vi "Video Stuff v03.vi"() -> ()   [LabVIEW 2009]
doc: "This example illustrates the use of a calibration grid to calibrate and correct an image for nonlinear distortion and accurate shape measurements.\n\nThis example loads the image of a calibration grid used to calibrate the system, learns the grid, then loads an image of parts acquired using the same setup. The example then corrects the image in two ways. The first method corrects the entire image and then measures the area of the coins. The second method corrects only the area of the coins and displays the difference in processing time."
uses:
  <vilib>/userDefined/High Color/IMAQdx.ctl
  <vilib>/vision/NI_Vision_Development_Module.lvlib
  <vilib>/vision/driver/NI_Vision_Acquisition_Software.lvlib
panel:
  out "Image Pixels (U8)":u8[][](array[numeric])
  out "Array":i32[][](array[numeric])
  in  "Overlay":bool
  out "Small":T1(plugin-control)
  in  "Resolution":i32=36
  in  "Color":u32(colorbox)=16711885
  in  "Pixel Coordinates":cluster{"X":sgl, "Y":sgl}={"X"=146.5, "Y"=183.95} {"Y" format="%.2f"; "X" format="%.2f"}
  out "Real World Coordinates":cluster{"X":sgl, "Y":sgl} {"Y" format="%.2f"; "X" format="%.2f"}
  out "Transform":T1(plugin-control)
  in  "Camera Name":T2="cam0"
  in  "Video Modes":i32(listbox)
  in  "stop":bool
  out "Live Video":T1(plugin-control)
  out "Buffer Number":u32
  out "Frame Rate":dbl(knob) scale=0.0..100.0 scale format="%.1f"
  in  "Red Range":cluster{"Lower value":i32, "Upper value":i32}={"Lower value"=240, "Upper value"=255}
  in  "Green Range":cluster{"Lower value":i32, "Upper value":i32}={"Lower value"=250, "Upper value"=255}
  in  "Blue Range":cluster{"Lower value":i32, "Upper value":i32}={"Lower value"=250, "Upper value"=255}
  in  "Color Mode":u16(ring) items=["RGB", "HSL", "HSV", "HSI"]
  out "Super Filter":T1(plugin-control)
  in  "Calibration File Path":path=path "C:/Documents and Settings/ekolker/My Documents/OGRE/to be synched/calibrationGrid.PNG"
  out "Top Image":T1(plugin-control) caption="Calibration Template"
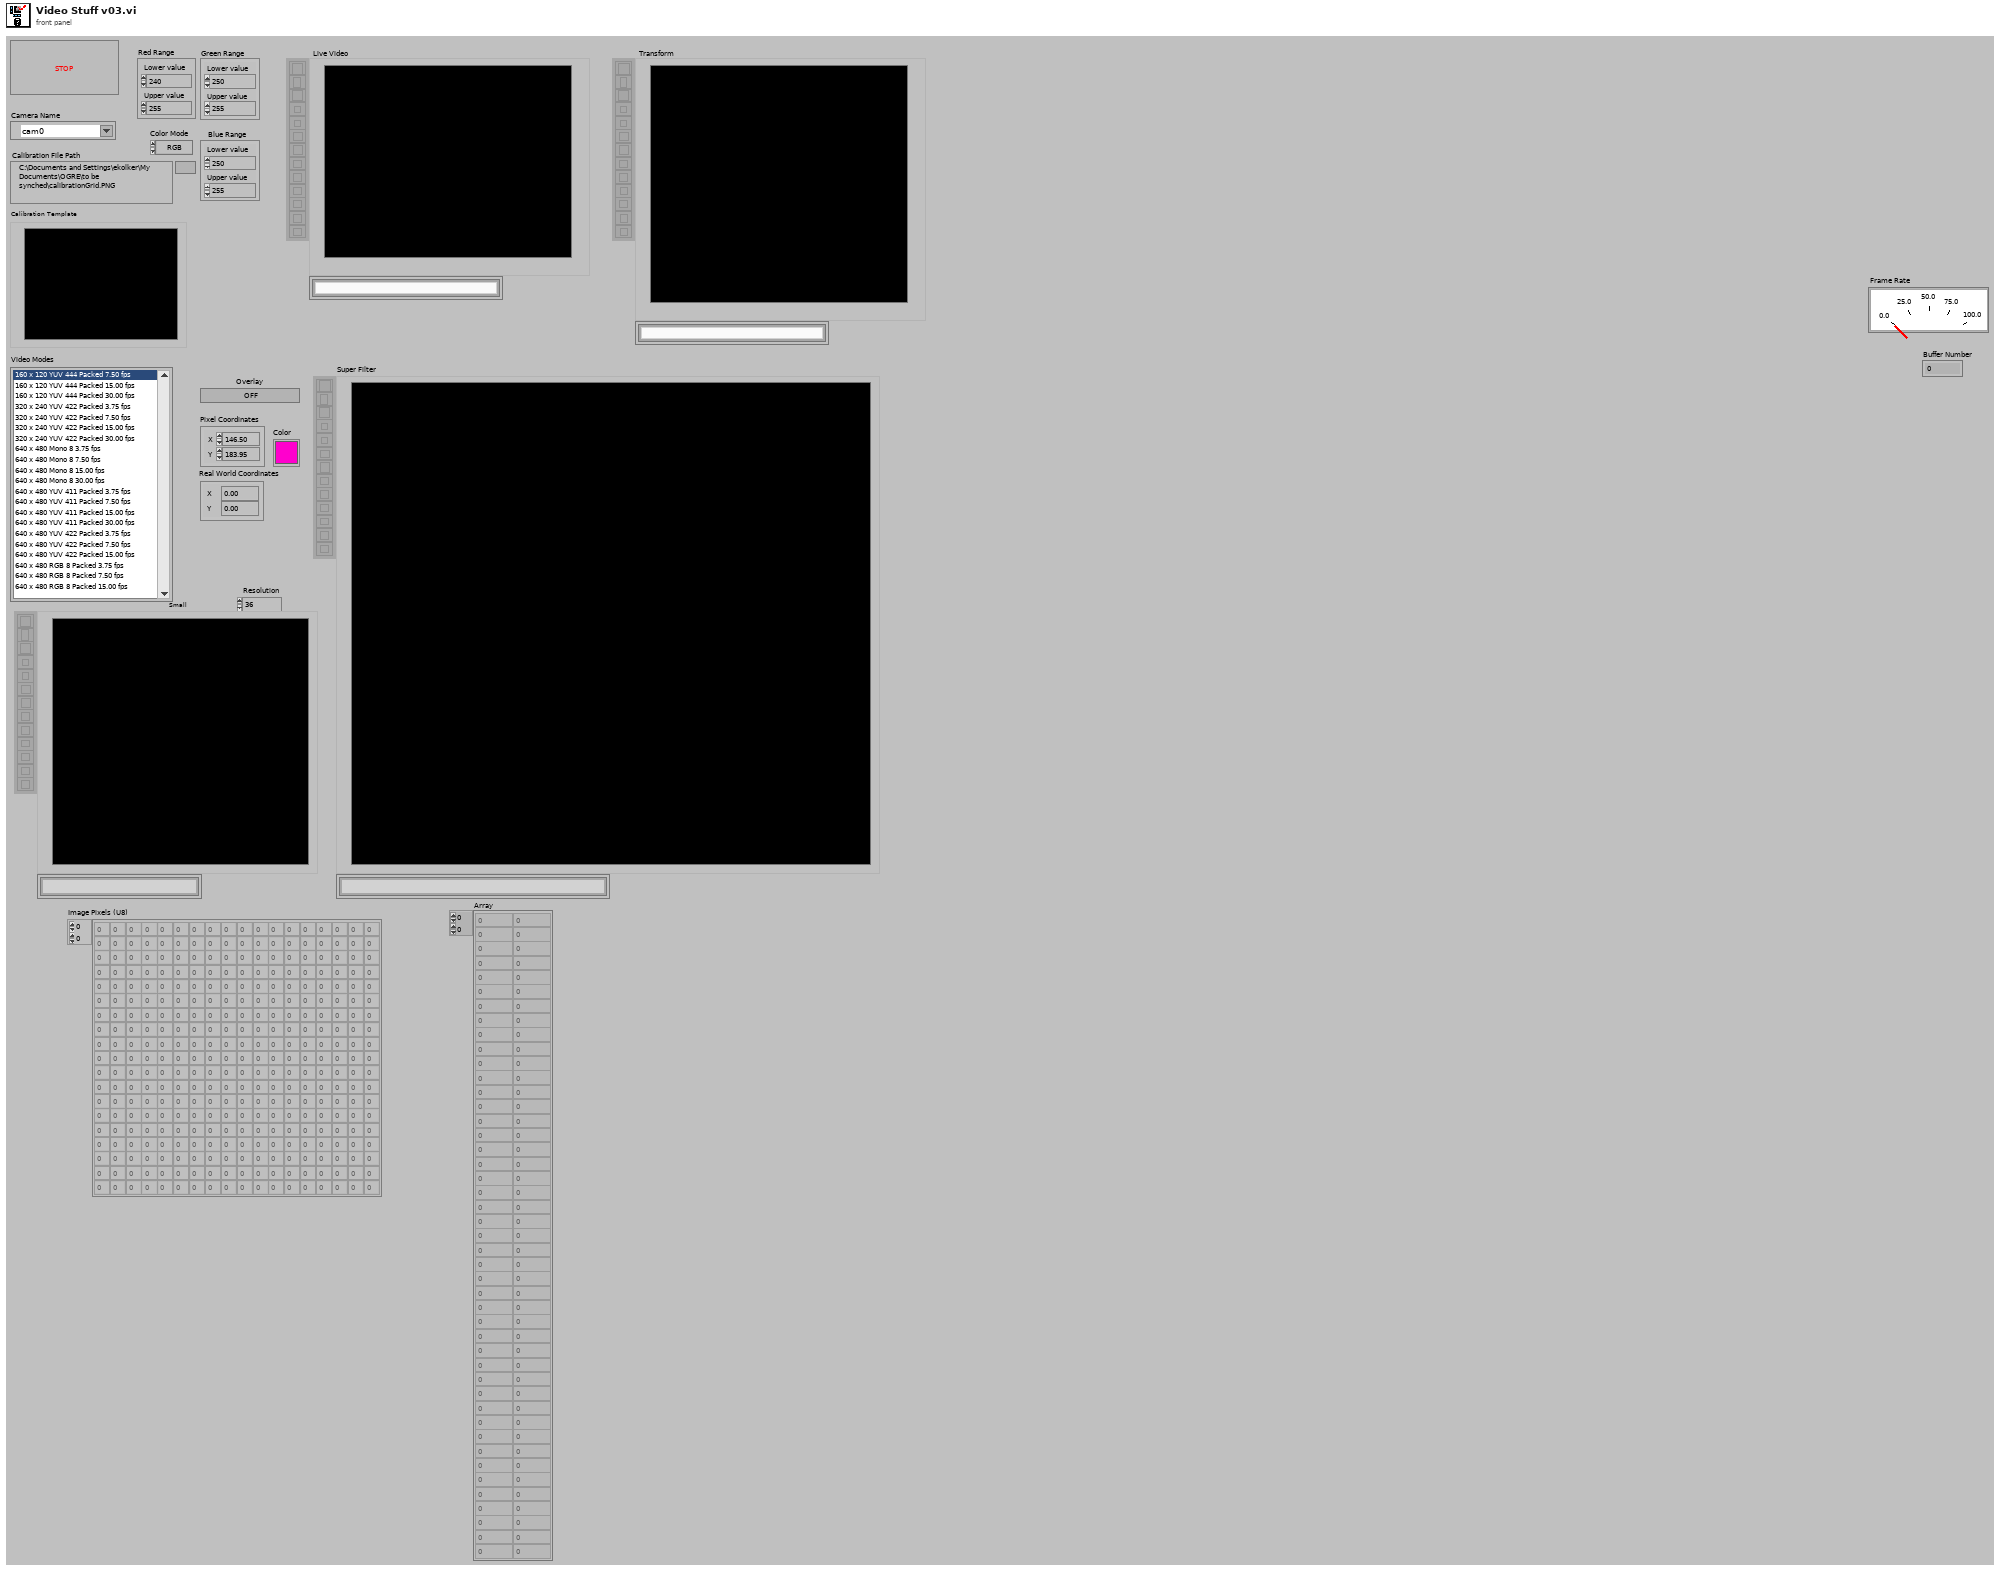
[diagram p1: front panel]
types:
  T1 = typedef "IMAQ Image.ctl" = refnum<image>
  T2 = typedef "IMAQdx.ctl" = refnum<k21>
  T3 = typedef "Image Type" = u32
  T4 = cluster{"X Step":sgl, "Y Step":sgl, "Unit":u32, "Threshold Range":cluster{"Lower value":sgl, "Upper value":sgl}}
  T5 = cluster{"Distortion":u32, "Corrected Image Scaling":u32, "Corrected Image Learn ROI":u32, "Learn Error Map?":bool, "Learn Correction Table?":bool}
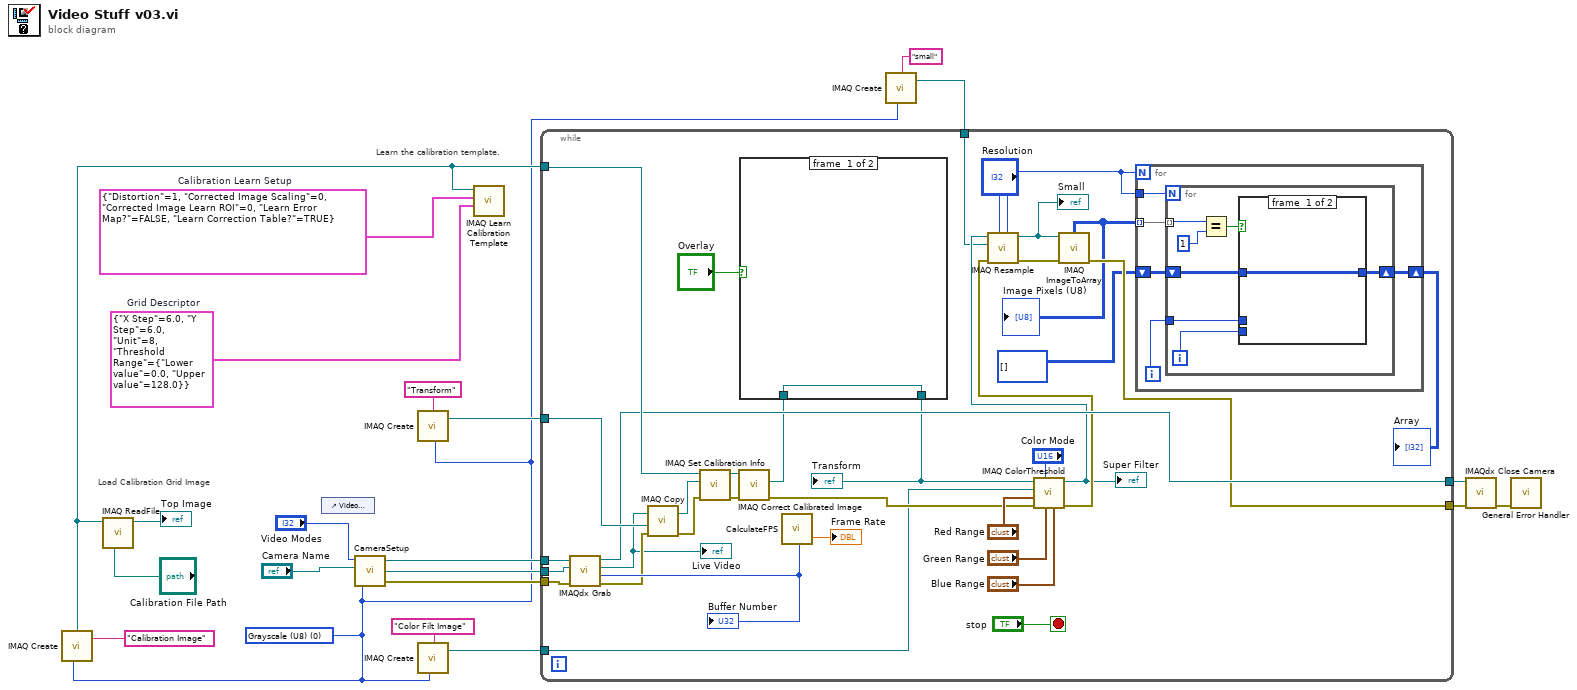
[diagram p0: block diagram]
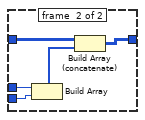
[diagram p2: hidden frame]
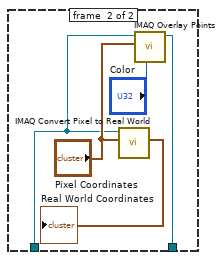
[diagram p3: hidden frame]
diagram:
  w1 = T3 0 items=["Grayscale (U8)", "Grayscale (I16)", "Grayscale (SGL)", "Complex (CSG)", "RGB (U32)", "HSL (U32)", "RGB (U64)", "Grayscale (U16)"] ("Image Type")
  w15 = T4 {"X Step"=6.0, "Y Step"=6.0, "Unit"=8, "Threshold Range"={"Lower value"=0.0, "Upper value"=128.0}}  # Grid Descriptor
  w16 = T5 {"Distortion"=1, "Corrected Image Scaling"=0, "Corrected Image Learn ROI"=0, "Learn Error Map?"=FALSE, "Learn Correction Table?"=TRUE}  # Calibration Learn Setup
  # "Load Calibration Grid Image"
  # "Learn the calibration template."
  n1 = call "IMAQ Create"("Image Name"="Calibration Image", "Image Type"=w1) -> ("New Image"=w21:T1)  [unwired: 2 in, 2 out]
  n2 = call "IMAQ ReadFile"("File Path"="Calibration File Path", "Image"=w21) -> ("Image Out"=→"Top Image":T1)  [unwired: 3 in, 6 out]
  n3 = control-ref of="Video Modes"() -> ()  [unwired: 1 out]
  n4 = call "CameraSetup.vi"("Image Type"=w1, "Camera Name"="Camera Name", "Video Modes"="Video Modes") -> ("error out"=w9:errorcluster, "New Image"=w4:T1, "Session Out"=w5:T2)  [unwired: 1 in]
  n5 = call "IMAQ Create"("Image Name"="Transform", "Image Type"=w1) -> ("New Image"=w17:T1)  [unwired: 2 in, 2 out]
  n6 = call "IMAQ Create"("Image Name"="Color Filt Image", "Image Type"=w1) -> ("New Image"=w18:T1)  [unwired: 2 in, 2 out]
  n7 = call "IMAQ Learn Calibration Template"("Grid Descriptor"=w15, "Calibration Learn Setup"=w16, "Image"=w21) -> ()  [unwired: 4 in, 5 out]
  n8 = call "IMAQ Create"("Image Name"="small", "Image Type"=w1) -> ("New Image"=w7:T1)  [unwired: 2 in, 2 out]
  n9 = while {
    tunnel: w21 -> [w47]
    tunnel: w18 -> [w35]
    tunnel: [w44] -> w19
    tunnel: w17 -> [w45]
    tunnel: w9 -> [w37]
    tunnel: w7 -> [w31]
    tunnel: [w25] -> w6
    tunnel: w5 -> [w30]
    tunnel: w4 -> [w29]
    stop <- "stop" stop-if-true
    n10 = call <vilib>:"IMAQdx Grab.vi"("error in"=w37, "Image In"=w29, "Session In"=w30) -> ("error out"=w38:errorcluster, "Buffer Number Out"=w49:u32, "Image Out"=w34:T1, "Session Out"=w44:T2)  [unwired: 1 in, 4 out]
    "Live Video" <- w34
    "Buffer Number" <- w49
    n11 = call "IMAQ Copy"("error in (no error)"=w38, "Image Dst"=w45, "Image Src"=w34) -> ("error out"=w39:errorcluster, "Image Dst Out"=w48:T1)  [unwired: 3 in]
    n12 = call "IMAQ Set Calibration Info"("error in (no error)"=w39, "Image Dst"=w48, "Image Src"=w47) -> ("error out"=w40:errorcluster, "Calibrated Image"=w46:T1)  [unwired: 1 in, 6 out]
    n13 = call "IMAQ Correct Calibrated Image"("error in (no error)"=w40, "Image Src"=w46) -> ("error out"=w41:errorcluster, "Corrected Image"=w43:T1)  [unwired: 5 in, 3 out]
    n14 = case shown="False" "Overlay" {
      tunnel: w43 -> [w74 w77]
      tunnel: [w74 w76] -> w42
      frame #0 {
      }
      frame #1 {
        n15 = call "IMAQ Convert Pixel to Real World"("Pixel Coordinates"="Pixel Coordinates", "Calibrated Image"=w77) -> ("Real World Coordinates"=→"Real World Coordinates":cluster{"X":sgl, "Y":sgl})  [unwired: 4 in, 5 out]
        n16 = call "IMAQ Overlay Points"("Color"="Color", "Point"="Pixel Coordinates", "Image"=w77) -> ("Image Out"=w76:T1)  [unwired: 7 in, 1 out]
      }
    }
    "Transform" <- w42
    n17 = call "CalculateFPS.vi"("buffer number"=w49) -> ("processed FPS"=→"Frame Rate":dbl)  [unwired: 2 out]
    n18 = call "IMAQ ColorThreshold"("Blue or Luma or Val or Inten Range"="Blue Range", "Green or Sat Range"="Green Range", "Color Mode"="Color Mode", "error in (no error)"=w41, "Red or Hue Range"="Red Range", "Image Dst"=w35, "Image Src"=w42) -> ("error out"=w33:errorcluster, "Image Dst Out"=w32:T1)  [unwired: 3 in]
    "Super Filter" <- w32
    n19 = call "IMAQ Resample"("X Resolution"="Resolution", "Y Resolution"="Resolution", "error in (no error)"=w33, "Image Dst"=w31, "Image Src"=w32) -> ("error out"=w28:errorcluster, "Image Dst Out"=w27:T1)  [unwired: 5 in]
    "Small" <- w27
    n20 = call "IMAQ ImageToArray"("error in (no error)"=w28, "Image"=w27) -> ("error out"=w25:errorcluster, "Image Pixels (U8)"=w24:u8[][])  [unwired: 2 in, 3 out]
    "Image Pixels (U8)" <- w24
    n21 = for {
      N: "Resolution" -> [_]
      tunnel: "Resolution" -> [w60]
      tunnel: w24 -> [w59] mode=indexing
      shift-right: [w58] -> w23
      shift-left: i32[][] [] -> [w57]
      i -> [w56]
      n22 = for {
        N: w60 -> [_]
        tunnel: w59 -> [w67] mode=indexing
        shift-right: [w65] -> w58
        shift-left: w57 -> [w62]
        tunnel: w56 -> [w63]
        i -> [w64]
        n23 = Equal?(x=w67, y=u8 1) -> (x = y?=w61:bool)
        n24 = case shown="True" w61 {
          tunnel: [w68 w73] -> w65
          tunnel: w64 -> [_ w72]
          tunnel: w63 -> [_ w71]
          tunnel: w62 -> [w68 w69]
          frame #0 {
          }
          frame #1 {
            n25 = Build Array(w71, w72) -> (w70:i32[])
            n26 = Build Array (concatenate)(w69, w70) -> (w73:i32[][])
          }
        }
      }
    }
    "Array" <- w23
  }
  n27 = call <vilib>:"IMAQdx Close Camera.vi"("error in"=w6, "Session In"=w19) -> ("error out"=w20:errorcluster)  [unwired: 9 out]
  n28 = call <vilib>:"General Error Handler.vi"("error in (no error)"=w20) -> ()  [unwired: 1 in, 14 out]
